vi "Get Current Step.vi"(8 "error in (no error)":errorcluster, 11 "Tester in":refnum<class "Tester.lvclass">) -> (0 "error out":errorcluster, 2 "Current Step":refnum<class "Step.lvclass">, 3 "Tester out":refnum<class "Tester.lvclass">)   [LabVIEW 2020, in "Tester.lvlib" / "Tester.lvclass"]
uses:
  Tester.lvclass
  Step/Step.lvclass
  Tester.lvclass/Tester.ctl
  Sequence/Sequence.lvclass
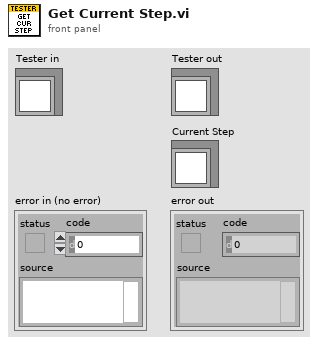
[diagram p1: front panel]
types:
  T1 = typedef "Tester.lvlib/Tester.lvclass/Execution Ref.ctl" = cluster{"Sequence":refnum<class "Sequence.lvclass">, "Step":i32, "Results":refnum<class "Results.lvclass">, "State":T2, "Run Step VI":refnum<vi>, "Abort":bool}
  T2 = typedef "Tester.lvlib/Tester.lvclass/State.ctl" = enum16{"Idle", "In Progress", "Completed"}
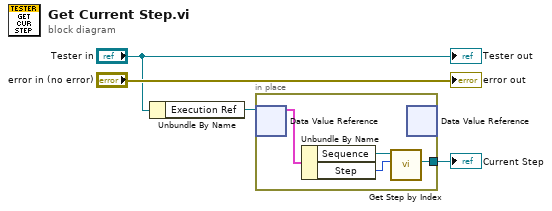
[diagram p0: block diagram]
diagram:
  n1 = Unbundle By Name("Tester in") -> ("Execution Ref"=w3:refnum<data-value>)
  n2 = in-place {
    in-place-border: [w5] -> w1
    n3 = in-place-dvr #1(w3) -> (w8:T1)  [unwired: 1 out]
    n4 = Unbundle By Name(w8) -> ("Sequence"=w7:refnum<class "Sequence.lvclass">, "Step"=w6:i32)
    n5 = call "Get Step by Index.vi"("Step Index"=w6, "Sequence in"=w7) -> ("Step"=w5:refnum<class "Step.lvclass">)  [unwired: 7 in, 2 out]
    n6 = in-place-dvr #1() -> ()  [unwired: 1 in, 2 out]
  }
  "Current Step" <- w1
  "error out" <- "error in (no error)"
  "Tester out" <- "Tester in"
